vi "Main.vi"(11 "Module Admin":refnum<class "Delacor_lib_QMH_Module Admin.lvclass">) -> ()   [LabVIEW 2019, in "Tester UI.lvlib"]
doc: "This template is based off of the Queued Message Handler design pattern and the Queued Message Handler project template that ships with LabVIEW.\n\nThe main difference is that the queue is private to this module and communication between modules is performed via Broadcast and Request events.\n\nRequest events are wrapped in public API methods and are handled in the Event Handling Loop (EHL) of this VI. Any module can register for Broadcast events sent by this module. The EHL generates messages based on user interface actions.\n\nThe Message Handling Loop (MHL) processes messages generated by the EHL, or by other messages. The messages are string values, so new messages can be added easily to the Message Cases case structure in the MHL. Each message cluster can also provide an optional value for Message Data, which is a variant that can be converted to whatever message-specific data is required.\n_____\nBased on Delacor QMH Project Template 5.0.0.82."
uses:
  Tester UI.lvlib
  Module Data--cluster.ctl
  <vilib>/Delacor/Delacor QMH/Libraries/Message Queue_class/Delacor_lib_QMH_Message Queue.lvclass
  <vilib>/Delacor/Delacor QMH/Libraries/Message Queue_class/Delacor_lib_QMH_Enqueue Message (Single).vi
  <vilib>/ErrorRing/Error Ring.xnode
  <vilib>/Utility/error.llb/Error Cluster From Error Code.vi
  <vilib>/Delacor/Delacor QMH/Libraries/Module Admin_class/Delacor_lib_QMH_Module Admin.lvclass
  Stop Argument--cluster.ctl
  <vilib>/Utility/miscctls.llb/LVPointTypeDef.ctl
panel:
  out "Status":string
  out "error out":errorcluster
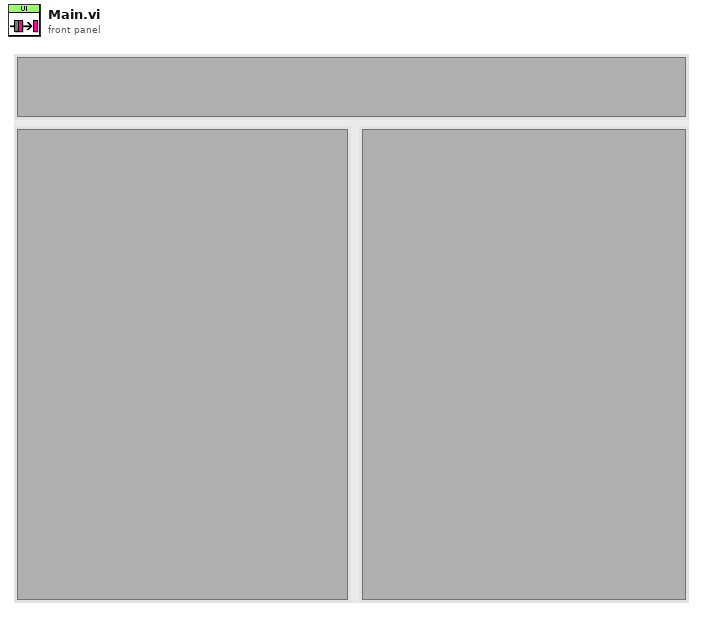
[diagram p1: front panel]
types:
  T1 = typedef "Tester UI.lvlib/Request Events--cluster.ctl" = cluster{"Stop Module":refnum<user-event>, "Show Panel":refnum<user-event>, "Hide Panel":refnum<user-event>, "Get Module Execution Status":refnum<user-event>, "Show Diagram":refnum<user-event>}
  T2 = typedef "Tester UI.lvlib/Module Data--cluster.ctl" = cluster{"Status":string}
  T3 = enum32{"invalid lock state", "Not Locked", "Locked (No Password)", "Password-protected"}
  T4 = typedef "Tester UI.lvlib/Stop Argument--cluster.ctl" = cluster{"Origin":string, "Exit via Stop Module Req?":bool, "Wait for Module to stop?":bool}
  T5 = enum32{"Invalid", "Standard", "Closed", "Hidden", "Minimized", "Maximized"}
  T6 = typedef "LVPointTypeDef.ctl" = cluster{"Horizontal":i16, "Vertical":i16}
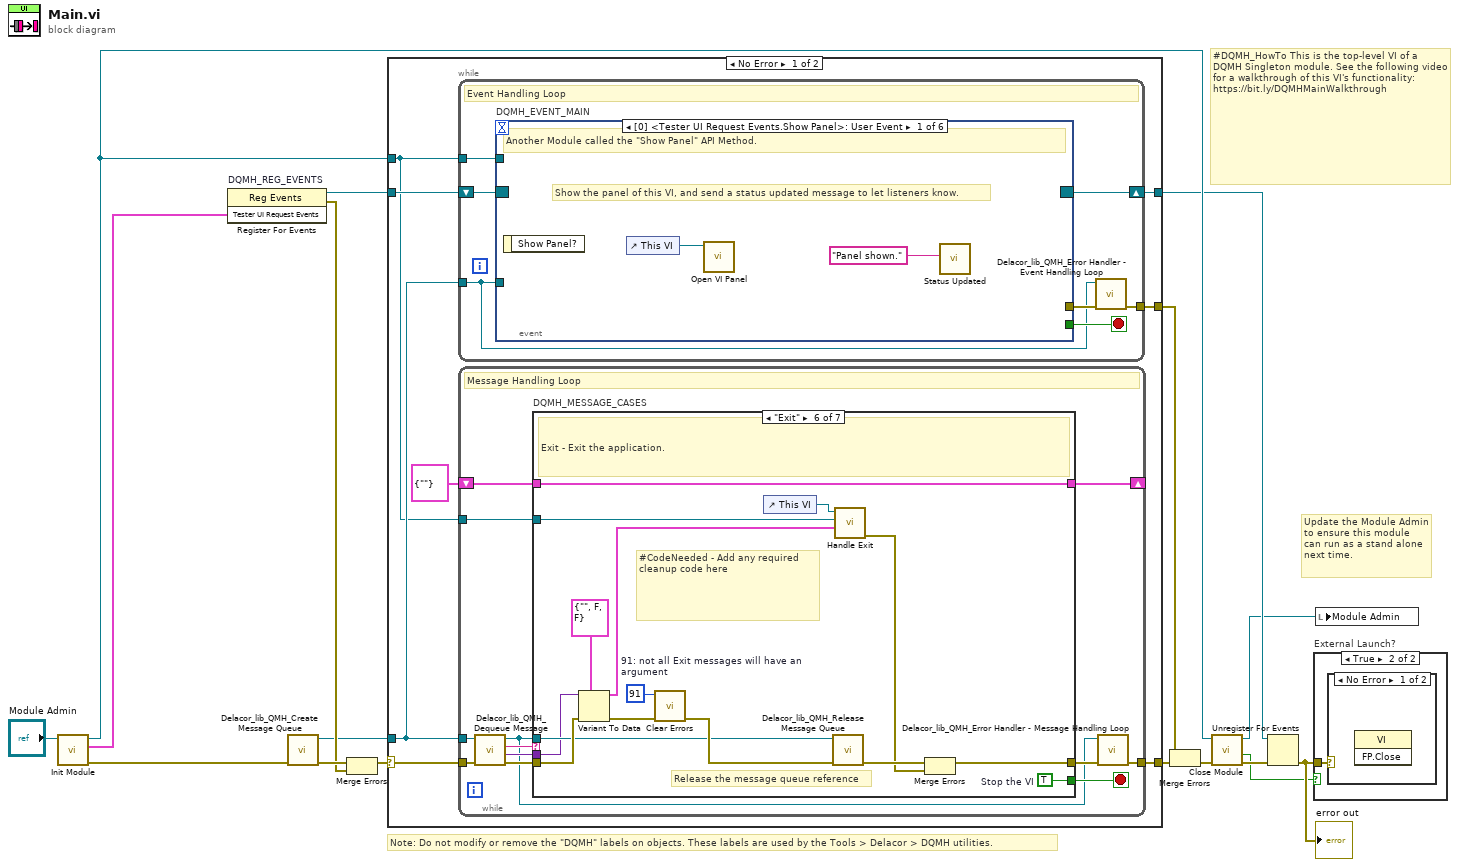
[diagram p0: block diagram]
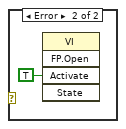
[diagram p3: hidden frame]
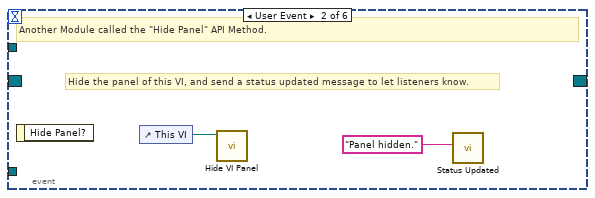
[diagram p4: hidden frame]
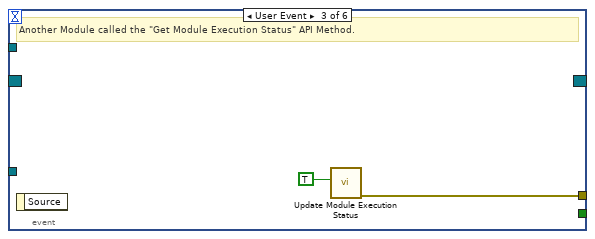
[diagram p5: hidden frame]
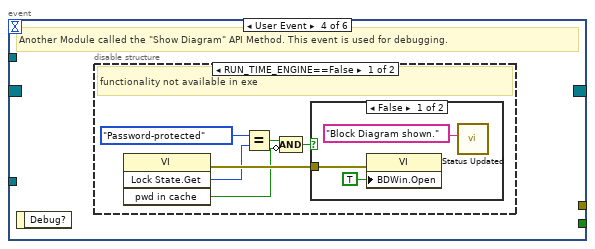
[diagram p6: hidden frame]
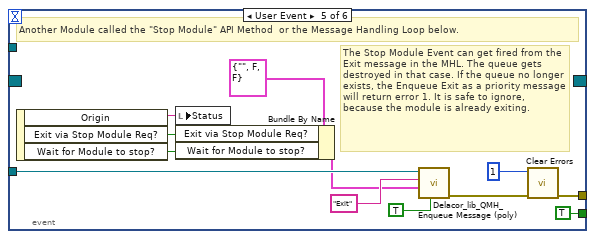
[diagram p9: hidden frame]
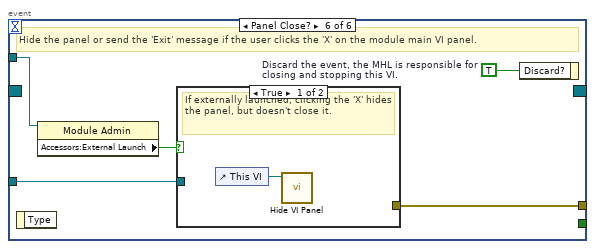
[diagram p10: hidden frame]
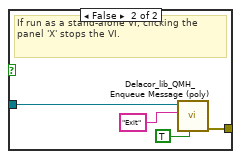
[diagram p11: hidden frame]
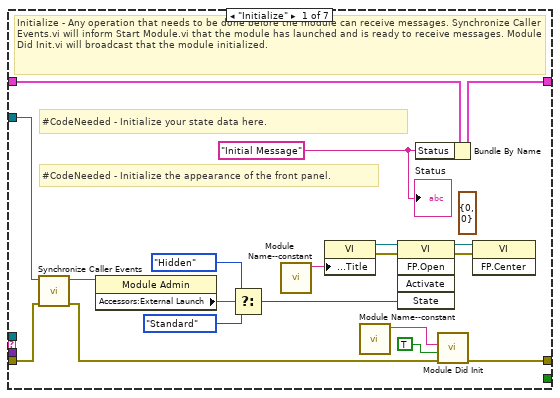
[diagram p12: hidden frame]
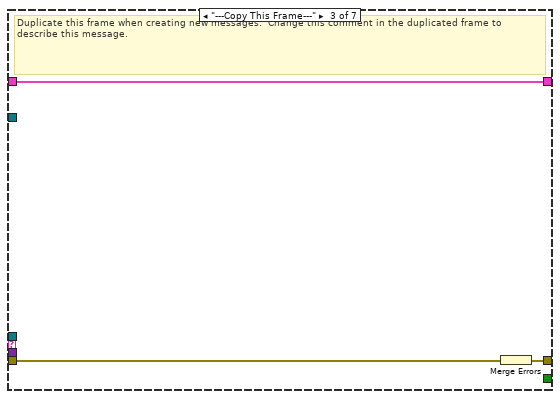
[diagram p14: hidden frame]
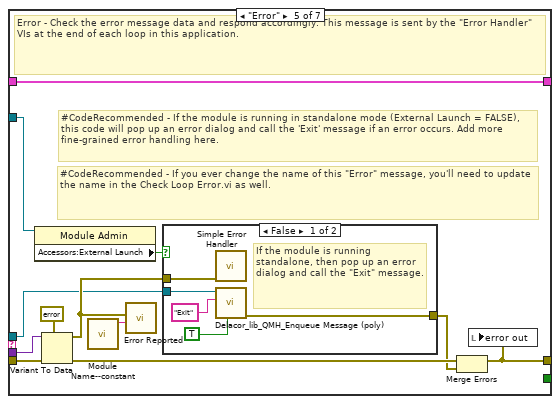
[diagram p16: hidden frame]
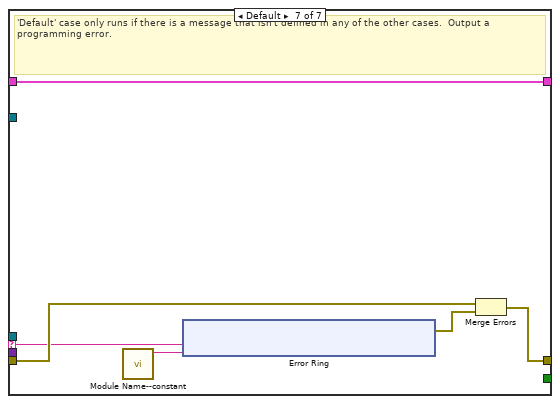
[diagram p18: hidden frame]
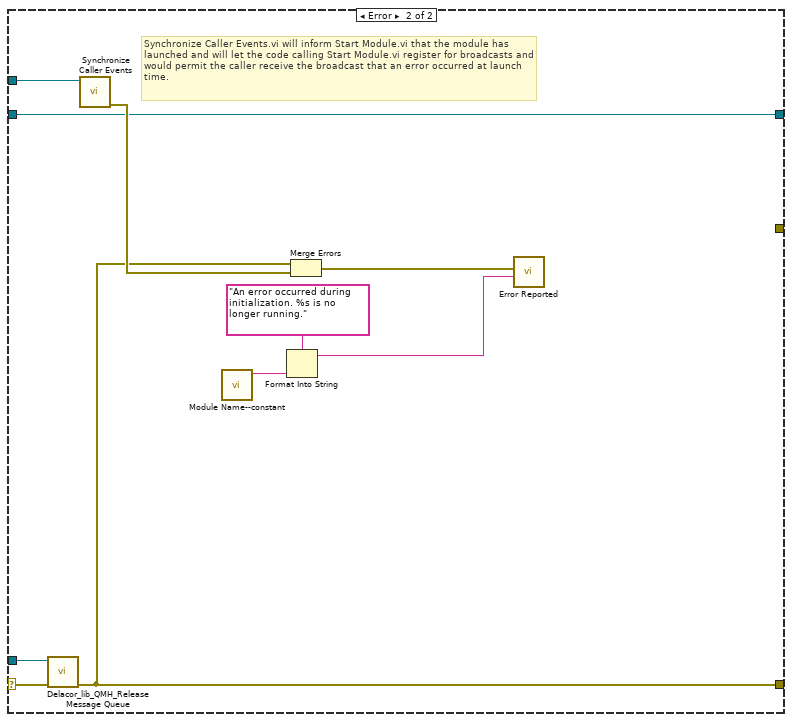
[diagram p19: hidden frame]
diagram:
  # "#DQMH_HowTo This is the top-level VI of a DQMH Singleton module. See the following video for a walkthrough of this VI's functionality: https://bit.ly/DQMHMainWalkthrough"
  # "Note: Do not modify or remove the \"DQMH\" labels on objects. These labels are used by the Tools > Delacor > DQMH utilities."
  # "Update the Module Admin to ensure this module can run as a stand alone next time."
  n1 = call "Init Module.vi"("Singleton Module Admin in"="Module Admin") -> ("error out"=w16:errorcluster, "Tester UI Request Events"=w5:T1, "Singleton Module Admin out"=w8:refnum<class "Delacor_lib_QMH_Module Admin.lvclass">)  [unwired: 8 in]
  n2 = register-events "DQMH_REG_EVENTS"(w5) -> (reference out=w6:refnum<event-registration>, error out=w9:errorcluster)  [unwired: 2 in]
  n3 = call <vilib>:"Delacor_lib_QMH_Create Message Queue.vi"("error in (no error)"=w16) -> ("error out"=w11:errorcluster, "Message Queue"=w4:refnum<class "Delacor_lib_QMH_Message Queue.lvclass">)  [unwired: 9 in]
  n4 = Merge Errors(w11, w9) -> (w10:errorcluster)
  n5 = case shown="No Error" w10 {
    selector: w10 -> [w23 w157]
    tunnel: [w25 w156] -> w17
    tunnel: [w22 w162] -> w7
    tunnel: w6 -> [w20 w162]
    tunnel: w4 -> [w19 w155]
    tunnel: [w24 _] -> w14
    tunnel: w8 -> [w18 w158]
    frame No Error {
      n6 = while {
        tunnel: w19 -> [w26]
        shift-right: [w29] -> w22
        shift-left: w20 -> [w30]
        tunnel: [w31] -> w24
        tunnel: w18 -> [w27]
        stop <- w28 stop-if-true
        # "Event Handling Loop"
        n7 = event "DQMH_EVENT_MAIN" shown="[0] <Tester UI Request Events.Show Panel>: User Event" {
          selector: w30 -> [_ _ _ _ _ _]
          dyn-events: [_ _ _ _ _ _] -> w29
          timeout: _ -> [_ _ _ _ _ _]
          tunnel: [_ _ _ _ TRUE ("Discard?") _] -> w28
          tunnel: w26 -> [_ _ _ _ w55 w62]
          tunnel: [_ _ w38 _ w58 w64] -> w32
          tunnel: w27 -> [_ _ _ _ _ w61]
          event User Event {
            # "Show the panel of this VI, and send a status updated message to let listeners know."
            # "Another Module called the \"Show Panel\" API Method."
            n8 = event-data() -> ()  [unwired: 1 in, 1 out]
            n9 = control-ref of="This VI"() -> (w34:refnum<vi>)
            n10 = call "Open VI Panel.vi"("VI"=w34) -> ()  [unwired: 10 in, 1 out]
            n11 = call "Status Updated.vi"("Status"="Panel shown." ("format string")) -> ()  [unwired: 10 in, 1 out]
          }
          event User Event {
            # "Hide the panel of this VI, and send a status updated message to let listeners know."
            # "Another Module called the \"Hide Panel\" API Method."
            n12 = event-data() -> ()  [unwired: 1 in, 1 out]
            n13 = control-ref of="This VI"() -> (w36:refnum<vi>)
            n14 = call "Hide VI Panel.vi"("VI"=w36) -> ()  [unwired: 10 in, 1 out]
            n15 = call "Status Updated.vi"("Status"="Panel hidden." ("format string")) -> ()  [unwired: 10 in, 1 out]
          }
          event User Event {
            # "Another Module called the \"Get Module Execution Status\" API Method."
            n16 = event-data() -> ()  [unwired: 1 in, 1 out]
            n17 = call "Update Module Execution Status.vi"("Running?"=TRUE) -> ("error out"=w38:errorcluster)  [unwired: 10 in]
          }
          event User Event {
            # "Another Module called the \"Show Diagram\" API Method. This event is used for debugging."
            n18 = event-data() -> ()  [unwired: 1 in, 1 out]
            n19 = disable-structure shown="RUN_TIME_ENGINE==False" {
              frame condition #0 (active) {
                # "functionality not available in exe"
                n20 = invoke class="VI" method="Lock State.Get"() -> (error out=w44:errorcluster, "Get Lock State"=w43:T3, "pwd in cache"=w40:bool)  [unwired: 4 in, 1 out]
                n21 = Equal?(x=T3."Password-protected", y=w43) -> (x = y?=w41:bool)
                n22 = Compound Arithmetic op=AND(w41, invert w40) -> (w39:bool)
                n23 = case shown="False" w39 {
                  tunnel: w44 -> [w47 _]
                  frame False {
                    n24 = property class="VI"(error in=w47, "BDWin.Open"=TRUE ("Block Diagram Window:Open")) -> ()  [unwired: 1 in, 2 out]
                    n25 = call "Status Updated.vi"("Status"="Block Diagram shown." ("format string")) -> ()  [unwired: 10 in, 1 out]
                  }
                  frame True {
                    # "Password-protected VI, and the password is not in the cache. Do not show the diagram."
                  }
                }
              }
              frame condition #1 {
              }
            }
          }
          event User Event {
            # "The Stop Module Event can get fired from the Exit message in the MHL. The queue gets destroyed in that case. If the queue no longer exists, the Enqueue Exit as a priority message will return error 1. It is safe to ignore, because the module is already exiting."
            # "Another Module called the \"Stop Module\" API Method  or the Message Handling Loop below."
            n26 = event-data() -> ("Origin"=w54:string, "Exit via Stop Module Req?"=w50:bool, "Wait for Module to stop?"=w49:bool)  [unwired: 1 in]
            n27 = local write "Status"(w54) -> ()
            n28 = Bundle By Name(cluster=T4 {"Origin"="", "Exit via Stop Module Req?"=FALSE, "Wait for Module to stop?"=FALSE} ("Stop Argument"), "Exit via Stop Module Req?"=w50, "Wait for Module to stop?"=w49) -> (w48:T4)
            n29 = call-poly <vilib>:"Delacor_lib_QMH_Enqueue Message (poly).vi"("Priority Message? (F)"=TRUE, "Message Data"=w48, "Message"="Exit", "Message Queue in"=w55) -> ("error out"=w59:errorcluster)  [unwired: 6 in, 1 out]
            n30 = call <vilib>:"Clear Errors.vi"("error in (no error)"=w59, "specific error code to clear (0: all)"=1) -> ("error out"=w58:errorcluster)  [unwired: 4 in, 1 out]
          }
          event Panel Close? {
            w63 = TRUE  # Discard the event, the MHL is responsible for closing and stopping this VI.
            # "Hide the panel or send the 'Exit' message if the user clicks the 'X' on the module main VI panel."
            n31 = event-data() -> ()  [unwired: 1 in, 1 out]
            n32 = property class="Module Admin"(reference=w61) -> ("Accessors:External Launch"=w60:bool)  [unwired: 1 in, 2 out]
            n33 = case shown="True" w60 {
              tunnel: w62 -> [_ w68]
              tunnel: [_ w69] -> w64
              frame True {
                # "If externally launched, clicking the 'X' hides the panel, but doesn't close it."
                n34 = control-ref of="This VI"() -> (w65:refnum<vi>)
                n35 = call "Hide VI Panel.vi"("VI"=w65) -> ()  [unwired: 10 in, 1 out]
              }
              frame False {
                # "If run as a stand-alone VI, clicking the panel 'X' stops the VI."
                n36 = call-poly <vilib>:"Delacor_lib_QMH_Enqueue Message (poly).vi"("Priority Message? (F)"=TRUE, "Message"="Exit", "Message Queue in"=w68) -> ("error out"=w69:errorcluster)  [unwired: 7 in, 1 out]
              }
            }
            n37 = event-data("Discard?"=w63) -> ()  [unwired: 1 in, 1 out]
          }
        }
        n38 = call-dynamic "Delacor_lib_QMH_Error Handler - Event Handling Loop.vi"("error in (no error)"=w32, "Message Queue in"=w26) -> ("dup error in"=w31:errorcluster)  [unwired: 8 in, 1 out]
      }
      n39 = while {
        tunnel: w19 -> [w72]
        shift-right: [w76] -> _
        shift-left: T2 {"Status"=""} ("Data Cluster") -> [w77]
        tunnel: w23 -> [w80]
        tunnel: [w78] -> w25
        tunnel: w18 -> [w70]
        stop <- w75 stop-if-true
        # "Message Handling Loop"
        n40 = call-dynamic "Delacor_lib_QMH_Dequeue Message.vi"("error in (no error)"=w80, "Message Queue in"=w72) -> ("error out"=w79:errorcluster, "Message Data"=w73:variant, "Message"=w74:string, "Message Queue out"=w71:refnum<class "Delacor_lib_QMH_Message Queue.lvclass">)  [unwired: 6 in]
        n41 = case "DQMH_MESSAGE_CASES" shown="\"Exit\"" w74 {
          selector: w74 -> [_ _ _ _ _ _ w142]
          tunnel: w71 -> [_ _ _ _ w112 w134 _]
          tunnel: w79 -> [w99 w103 w106 w108 w119 w140 w144]
          tunnel: [w97 w103 w105 w108 w115 w137 w145] -> w81
          tunnel: w77 -> [w88 w102 w104 w107 w114 w133 w143]
          tunnel: [w87 w102 w104 w107 w114 w133 w143] -> w76
          tunnel: [_ _ _ _ _ w132 _] -> w75
          tunnel: w73 -> [_ _ _ _ w113 w131 _]
          tunnel: w70 -> [w89 _ _ _ w111 w126 _]
          frame "Initialize" {
            w83 = T6 {"Horizontal"=0, "Vertical"=0} ("Origin")
            w82 = "Initial Message" ("Initial Message")
            # "#CodeNeeded - Initialize the appearance of the front panel."
            # "#CodeNeeded - Initialize your state data here."
            # "Initialize - Any operation that needs to be done before the module can receive messages. Synchronize Caller Events.vi will inform Start Module.vi that the module has launched and is ready to receive messages. Module Did Init.vi will broadcast that the module initialized."
            n42 = call "Synchronize Caller Events.vi"("error in (no error)"=w99, "Singleton Module Admin in"=w89) -> ("error out"=w98:errorcluster, "Singleton Module Admin out"=w84:refnum<class "Delacor_lib_QMH_Module Admin.lvclass">)  [unwired: 8 in]
            n43 = property class="Module Admin"(reference=w84) -> ("Accessors:External Launch"=w93:bool)  [unwired: 1 in, 2 out]
            n44 = Select(t=T5."Hidden" ("State"), s=w93, f=T5."Standard" ("State")) -> (s? t:f=w90:T5)
            n45 = call "Module Name--constant.vi"() -> ("Module Name"=w96:string)  [unwired: 11 in]
            n46 = property class="VI"("Front Panel.Title"=w96) -> (reference out=w95:refnum<vi>, error out=w101:errorcluster)  [unwired: 2 in]
            n47 = call "Module Name--constant.vi"() -> ("Module Name"=w85:string)  [unwired: 11 in]
            n48 = invoke class="VI" method="FP.Open"(reference=w95, error in=w101, "State"=w90) -> (reference out=w94:refnum<vi>, error out=w100:errorcluster)  [unwired: 2 in, 3 out]
            n49 = Bundle By Name(cluster=w88, "Status"=w82) -> (w87:T2)
            n50 = call "Module Did Init.vi"("error in (no error)"=w98, "Initialized?"=TRUE, "Origin"=w85) -> ("error out"=w97:errorcluster)  [unwired: 8 in]
            n51 = invoke class="VI" method="FP.Center"(reference=w94, error in=w100) -> ()  [unwired: 1 in, 3 out]
            "Status" <- w82
          }
          frame "--- Module Specific ---" {
            # "Separator -- The following cases handle messages specific to this Module."
          }
          frame "---Copy This Frame---" {
            # "Duplicate this frame when creating new messages.  Change this comment in the duplicated frame to describe this message."
            n52 = Merge Errors(w106) -> (w105:errorcluster)
          }
          frame "--- Exit and Error Handling---" {
            # "Separator - The following cases handle errors and exit messages."
          }
          frame "Error" {
            # "#CodeRecommended - If you ever change the name of this \"Error\" message, you'll need to update the name in the Check Loop Error.vi as well."
            # "#CodeRecommended - If the module is running in standalone mode (External Launch = FALSE), this code will pop up an error dialog and call the 'Exit' message if an error occurs. Add more fine-grained error handling here."
            # "Error - Check the error message data and respond accordingly. This message is sent by the \"Error Handler\" VIs at the end of each loop in this application."
            n53 = property class="Module Admin"(reference=w111) -> ("Accessors:External Launch"=w110:bool)  [unwired: 1 in, 2 out]
            n54 = Variant To Data(error in=w119, type=errorcluster {"status"=FALSE, "code"=0, "source"=""} ("error constant"), Variant=w113) -> (data=w120:errorcluster, error out=w117:errorcluster)
            n55 = call "Module Name--constant.vi"() -> ("Module Name"=w109:string)  [unwired: 11 in]
            n56 = call "Error Reported.vi"("Additional Information"=w109, "Error"=w120) -> ()  [unwired: 9 in, 1 out]
            n57 = case shown="False" w110 {
              tunnel: [w125 _] -> w116
              tunnel: w112 -> [w123 _]
              tunnel: w120 -> [w124 _]
              frame False {
                # "If the module is running standalone, then pop up an error dialog and call the \"Exit\" message."
                n58 = call <vilib>:"Simple Error Handler.vi"("error in (no error)"=w124) -> ()  [unwired: 4 in, 5 out]
                n59 = call-poly <vilib>:"Delacor_lib_QMH_Enqueue Message (poly).vi"("Priority Message? (F)"=TRUE, "Message"="Exit", "Message Queue in"=w123) -> ("error out"=w125:errorcluster)  [unwired: 7 in, 1 out]
              }
              frame True {
                # "If the module was launched externally, calling the Error Reported broadcast VI is the only action performed by the \"Error\" message. The module's caller can then process the error appropriately."
              }
            }
            n60 = Merge Errors(w117, w116) -> (w115:errorcluster)
            n61 = local write "error out"(w115) -> ()
          }
          frame "Exit" {
            w130 = 91  # 91: not all Exit messages will have an argument
            w132 = TRUE  # Stop the VI
            # "Release the message queue reference"
            # "#CodeNeeded - Add any required cleanup code here"
            # "Exit - Exit the application."
            n62 = Variant To Data(error in=w140, type=T4 {"Origin"="", "Exit via Stop Module Req?"=FALSE, "Wait for Module to stop?"=FALSE} ("Stop Argument"), Variant=w131) -> (data=w128:T4, error out=w136:errorcluster)
            n63 = call <vilib>:"Clear Errors.vi"("error in (no error)"=w136, "specific error code to clear (0: all)"=w130) -> ("error out"=w139:errorcluster)  [unwired: 4 in, 1 out]
            n64 = control-ref of="This VI"() -> (w127:refnum<vi>)
            n65 = call-dynamic "Delacor_lib_QMH_Release Message Queue.vi"("error in (no error)"=w139, "Message Queue"=w134) -> ("error out"=w138:errorcluster)  [unwired: 9 in]
            n66 = call "Handle Exit.vi"("Stop Argument"=w128, "Admin in"=w126, "VI reference"=w127) -> ("error out"=w135:errorcluster)  [unwired: 7 in, 1 out]
            n67 = Merge Errors(w138, w135) -> (w137:errorcluster)
          }
          frame Default {
            # "'Default' case only runs if there is a message that isn't defined in any of the other cases.  Output a programming error."
            n68 = call "Module Name--constant.vi"() -> ("Module Name"=w141:string)  [unwired: 11 in]
            n69 = xnode "Error Ring"("parameter 0"=w142, "parameter 1"=w141) -> ("error out"=w146:errorcluster)
            n70 = Merge Errors(w144, w146) -> (w145:errorcluster)
          }
        }
        n71 = call-dynamic "Delacor_lib_QMH_Error Handler - Message Handling Loop.vi"("error in (no error)"=w81, "Message Queue in"=w71) -> ("dup error in"=w78:errorcluster)  [unwired: 8 in, 1 out]
      }
    }
    frame Error {
      # "Synchronize Caller Events.vi will inform Start Module.vi that the module has launched and will let the code calling Start Module.vi register for broadcasts and would permit the caller receive the broadcast that an error occurred at launch time."
      n72 = call-dynamic "Delacor_lib_QMH_Release Message Queue.vi"("error in (no error)"=w157, "Message Queue"=w155) -> ("error out"=w156:errorcluster)  [unwired: 9 in]
      n73 = call "Synchronize Caller Events.vi"("Singleton Module Admin in"=w158) -> ("error out"=w163:errorcluster)  [unwired: 9 in, 1 out]
      n74 = call "Module Name--constant.vi"() -> ("Module Name"=w161:string)  [unwired: 11 in]
      n75 = Format Into String(format string="An error occurred during initialization. %s is no longer running.", w161) -> (resulting string=w159:string)  [unwired: 2 in, 1 out]
      n76 = Merge Errors(w156, w163) -> (w164:errorcluster)
      n77 = call "Error Reported.vi"("Additional Information"=w159, "Error"=w164) -> ()  [unwired: 9 in, 1 out]
    }
  }
  n78 = Merge Errors(w14, w17) -> (w13:errorcluster)
  n79 = call "Close Module.vi"("error in (no error)"=w13, "Module Admin in"=w8) -> ("error out"=w15:errorcluster, "External Launch"=w1:bool, "Module Admin out"=w2:refnum<class "Delacor_lib_QMH_Module Admin.lvclass">)  [unwired: 7 in]
  n80 = Unregister For Events(event registration refnum=w7, error in=w15) -> (error out=w12:errorcluster)
  "error out" <- w12
  n81 = case "External Launch?" shown="True" w1 {
    tunnel: w12 -> [_ w165]
    frame False {
    }
    frame True {
      n82 = case shown="No Error" w165 {
        frame No Error {
          n83 = invoke class="VI" method="FP.Close"() -> ()  [unwired: 3 in, 3 out]
        }
        frame Error {
          n84 = invoke class="VI" method="FP.Open"("Activate"=TRUE ("Activate?")) -> ()  [unwired: 4 in, 5 out]
        }
      }
    }
  }
  n85 = local write "Module Admin"(w2) -> ()
